vi "AppKind.vi"(11 "VI in":refnum<vi>) -> (3 "File Version Info":string)   [LabVIEW 2014]
uses:
  <vilib>/Utility/miscctls.llb/LVPointTypeDef.ctl
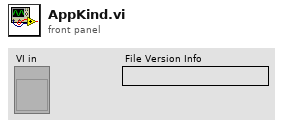
[diagram p1: front panel]
types:
  T1 = enum32{"invalid app kind", "Development System", "Run Time System", "Student Edition", "Embedded LabVIEW", "Evaluation", "Custom"}
  T2 = enum16{"Always On", "Always Off", "Off While Running"}
  T3 = enum32{"Invalid", "Standard", "Closed", "Hidden", "Minimized", "Maximized"}
  T4 = enum32{"Invalid", "Default", "Floating", "Floating/Auto-Hide", "Modal"}
  T5 = typedef "LVPointTypeDef.ctl" = cluster{"Horizontal":i16, "Vertical":i16}
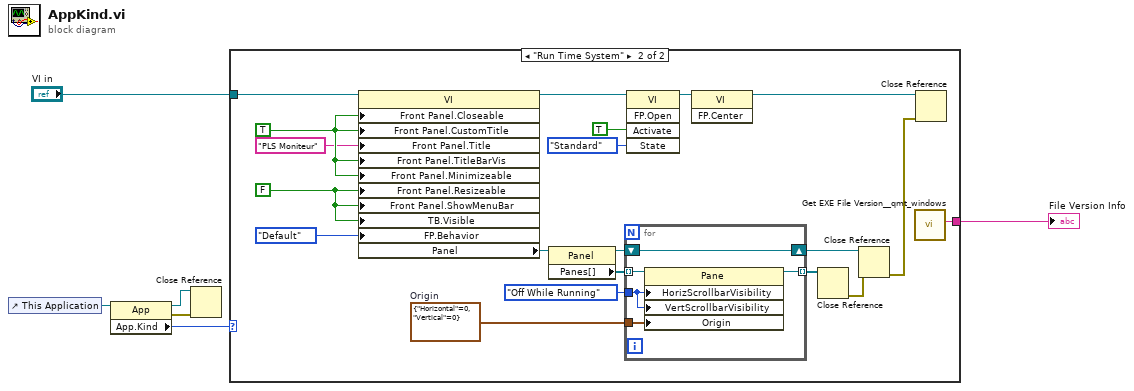
[diagram p0: block diagram]
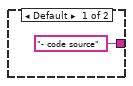
[diagram p2: hidden frame]
diagram:
  n1 = control-ref of="This Application"() -> (w1:refnum<vi>)
  n2 = property class="App"(reference=w1) -> (reference out=w3:refnum<vi>, error out=w4:errorcluster, "App.Kind"=w2:T1)  [unwired: 1 in]
  n3 = Close Reference(reference=w3, error in (no error)=w4) -> ()  [unwired: 1 out]
  n4 = case shown="\"Run Time System\"" w2 {
    tunnel: ["- code source" ("File Version Info") w9] -> w5
    tunnel: "VI in" -> [_ w8]
    frame Default {
    }
    frame "Run Time System" {
      w24 = T5 {"Horizontal"=0, "Vertical"=0}  # Origin
      w27 = TRUE
      w25 = FALSE
      n5 = property class="VI"(reference=w8, "Front Panel.Closeable"=w27, "Front Panel.CustomTitle"=w27, "Front Panel.Title"="PLS Moniteur" ("Front Panel Window:Title"), "Front Panel.TitleBarVis"=w27, "Front Panel.Minimizeable"=w27, "Front Panel.Resizeable"=w25, "Front Panel.ShowMenuBar"=w25, "TB.Visible"=w25, "FP.Behavior"=T4."Default") -> (reference out=w20:refnum<vi>, "Panel"=w18:refnum<vi>)  [unwired: 1 in, 1 out]
      n6 = property class="Panel"(reference=w18) -> (reference out=w15:refnum<vi>, "Panes[]"=w17:refnum<vi>[])  [unwired: 1 in, 1 out]
      n7 = for {
        tunnel: w17 -> [w32] mode=indexing
        tunnel: T2."Off While Running" -> [w31]
        shift-right: [w30] -> w12
        shift-left: w15 -> [w30]
        tunnel: [w29] -> w14 mode=indexing
        tunnel: w24 -> [w28]
        n8 = property class="Pane"(reference=w32, "HorizScrollbarVisibility"=w31, "VertScrollbarVisibility"=w31, "Origin"=w28) -> (reference out=w29:refnum<vi>)  [unwired: 1 in, 1 out]
      }
      n9 = invoke class="VI" method="FP.Open"(reference=w20, "Activate"=TRUE, "State"=T3."Standard") -> (reference out=w19:refnum<vi>)  [unwired: 2 in, 4 out]
      n10 = invoke class="VI" method="FP.Center"(reference=w19) -> (reference out=w10:refnum<vi>)  [unwired: 2 in, 2 out]
      n11 = Close Reference(reference=w14) -> (error out=w13:errorcluster)  [unwired: 1 in]
      n12 = Close Reference(reference=w12, error in (no error)=w13) -> (error out=w11:errorcluster)
      n13 = call <userlib>:"Get EXE File Version__qmt_windows.vi"() -> ("File Version Info"=w9:string)  [unwired: 9 in, 2 out]
      n14 = Close Reference(reference=w10, error in (no error)=w11) -> ()  [unwired: 1 out]
    }
  }
  "File Version Info" <- w5
